vi "main-inspection-project1.vi"() -> ()   [LabVIEW 2025]
uses:
  StateVariable.ctl
panel:
  in  "stop":bool
  out "Eff (%)":dbl
  out "Part No.":i32
  out "Pass (OK)":i32
  out "MSG State":string
  out "Part result":bool
  out "Bottom Hole Pass":bool
  out "Top Hole Pass":bool
  out "Main Hole Pass":bool
  out "Distance Pass":bool
  out "Bottom Radius (Pixels)":dbl
  out "Top Radius (Pixels)":dbl
  out "Main Radius (Pixels)":dbl
  out "Distance (Clamp1)":sgl format="%.2f"
  out "appended path":path
  out "Image":T1(plugin-control)
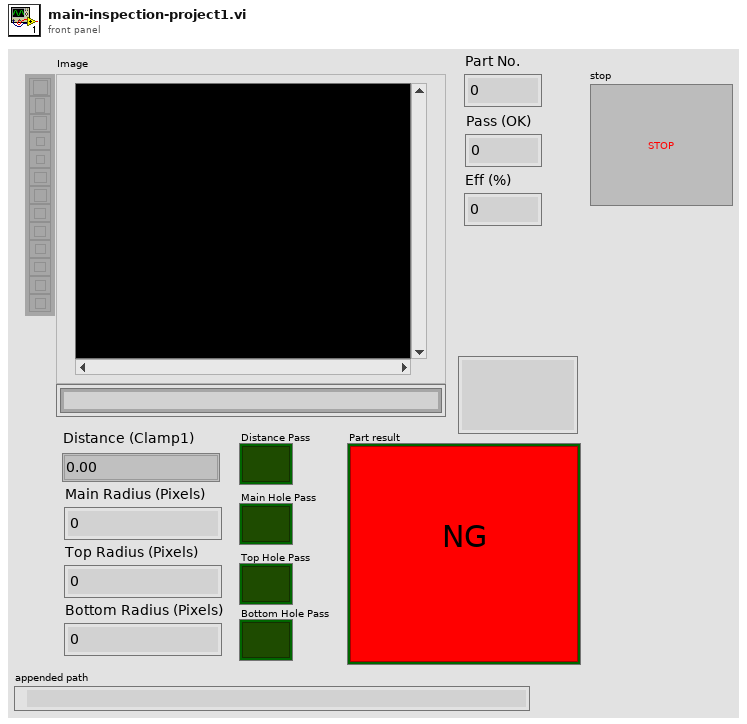
[diagram p1: front panel]
types:
  T1 = typedef "IMAQ Image.ctl" = refnum<image>
  T2 = cluster{"Distance (Clamp1)":sgl, "Main Radius (Pixels)":dbl, "Top Radius (Pixels)":dbl, "Bottom Radius (Pixels)":dbl, "Part result":bool, "Pass (OK)":i32, "PartNo.":i32, "Eff (%)":dbl, "refnum out":refnum<file>}
  T3 = typedef "StateVariable.ctl" = enum16{"Initialization", "Processing", "Checker", "Eff/Calc", "Logger", "Closed"}
  T4 = enum16{"open", "replace", "create", "open or create", "replace or create", "replace or create with confirmation"}
  T5 = cluster{"Center (Pixels)":cluster{"X":sgl, "Y":sgl}, "Radius (Pixels)":dbl, "Center (Real-World)":cluster{"X":sgl, "Y":sgl}, "Radius (Real-World)":dbl, "Roundness (Real-World)":dbl, "Average Strength":dbl, "Average SNR (dB)":dbl}
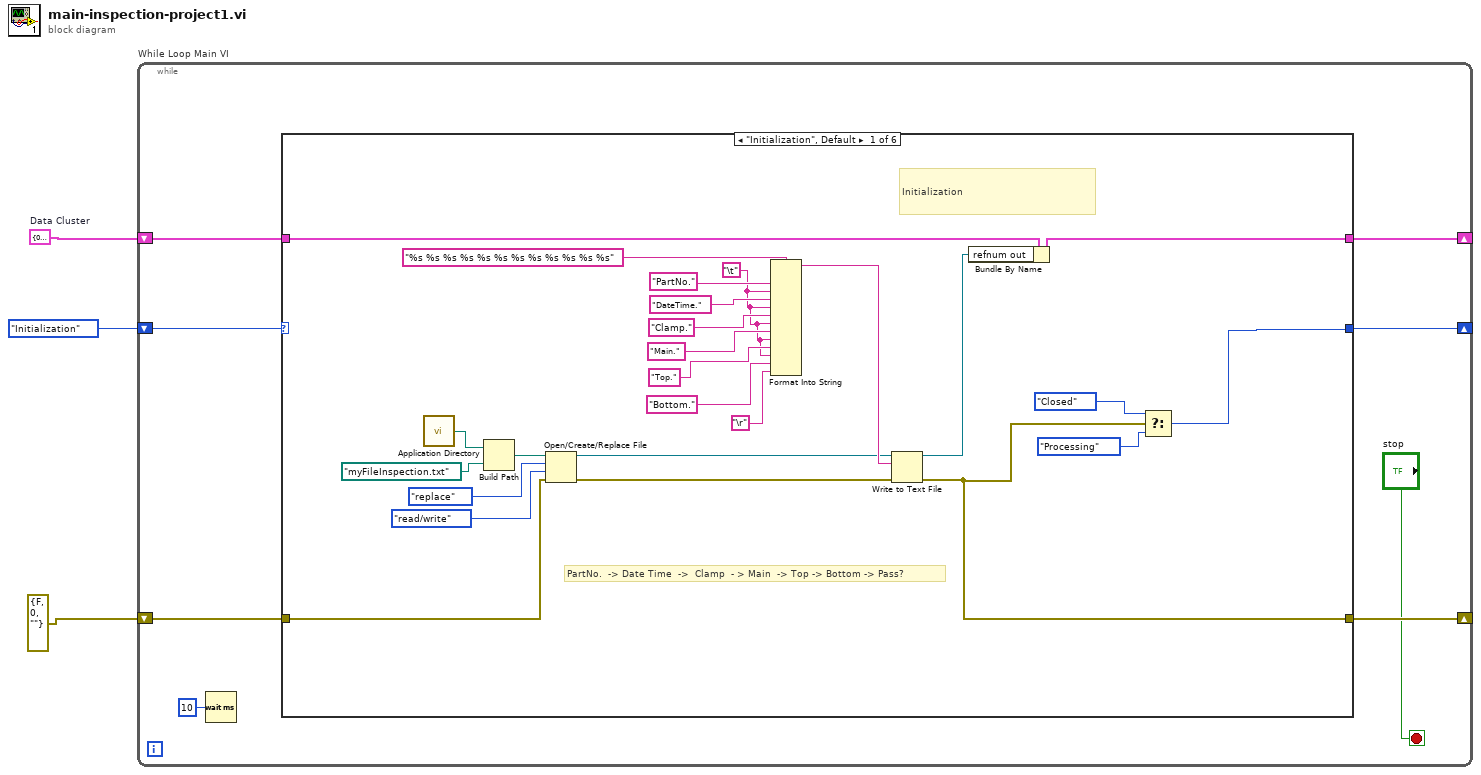
[diagram p0: block diagram]
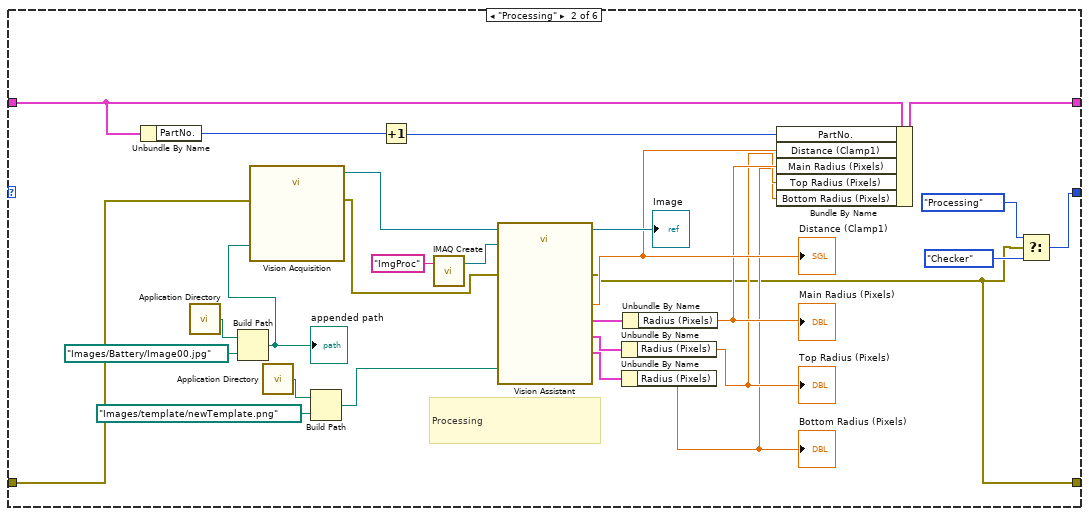
[diagram p2: hidden frame]
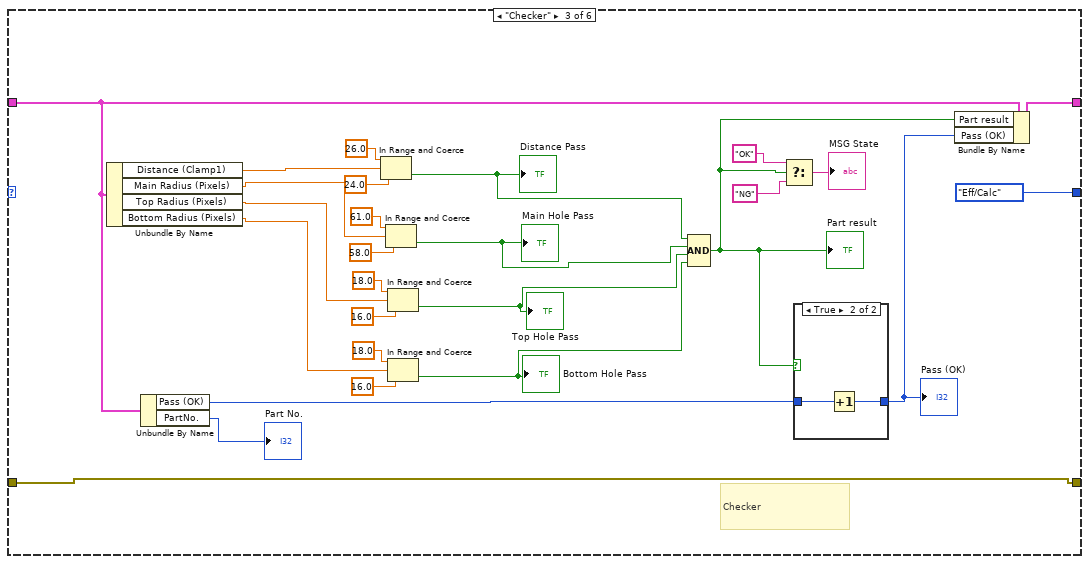
[diagram p3: hidden frame]
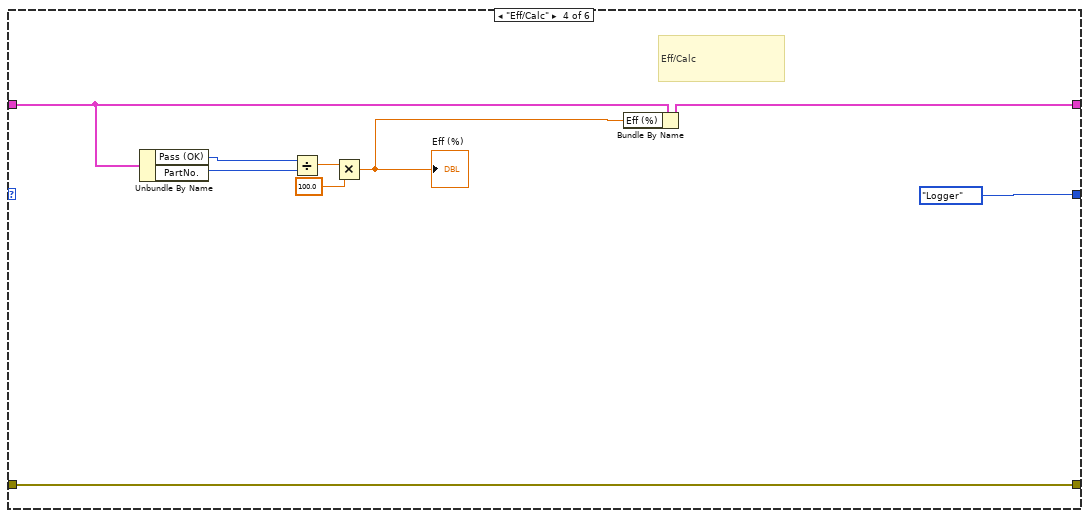
[diagram p5: hidden frame]
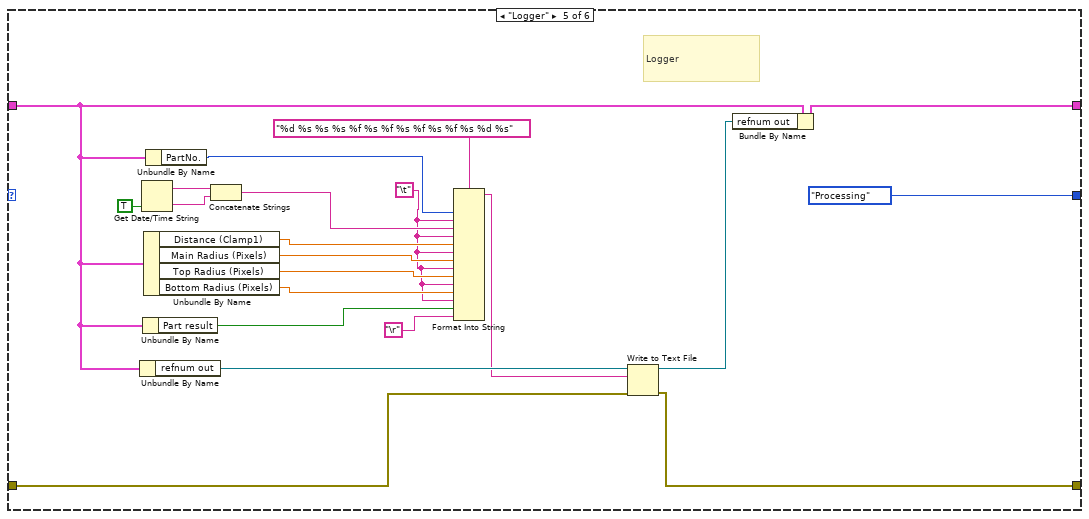
[diagram p6: hidden frame]
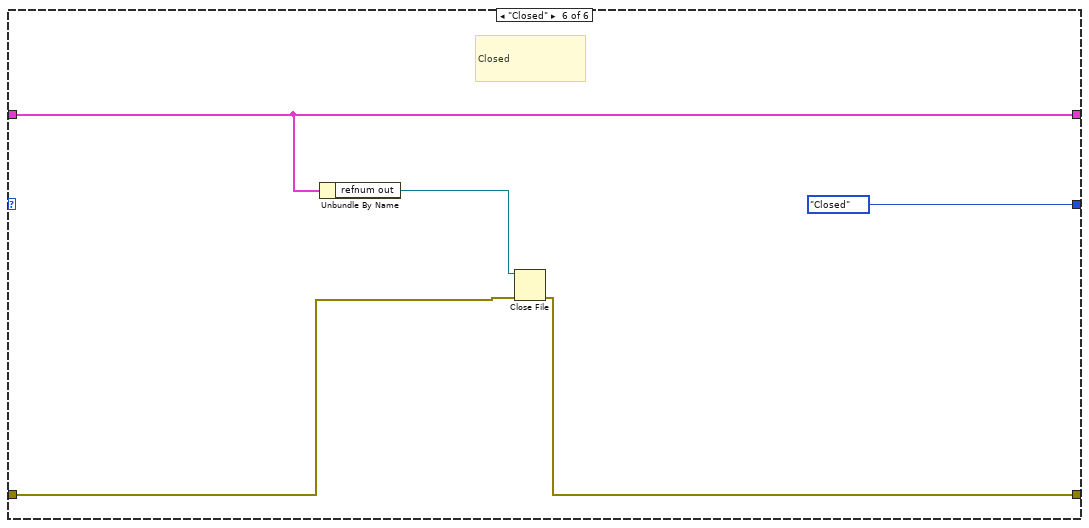
[diagram p7: hidden frame]
diagram:
  w2 = T2 {"Distance (Clamp1)"=0.0, "Main Radius (Pixels)"=0.0, "Top Radius (Pixels)"=0.0, "Bottom Radius (Pixels)"=0.0, "Part result"=FALSE, "Pass (OK)"=0, "PartNo."=0, "Eff (%)"=0.0, "refnum out"=refnum}  # Data Cluster
  n1 = while "While Loop Main VI" {
    shift-right: [w10] -> _
    shift-left: StateVariable."Initialization" ("Enum of State") -> [w11]
    shift-right: [w8] -> _
    shift-left: w2 -> [w9]
    shift-right: [w6] -> _
    shift-left: errorcluster {"status"=FALSE, "code"=0, "source"=""} ("error constant") -> [w7]
    stop <- "stop" stop-if-true
    n2 = Wait (ms)(milliseconds to wait=u32 10) -> ()  [unwired: 1 out]
    n3 = case shown="\"Initialization\", Default" w11 {
      tunnel: [w13 w40 StateVariable."Eff/Calc" ("Enum of State") StateVariable."Logger" ("Enum of State") StateVariable."Processing" ("Enum of State") StateVariable."Closed" ("Enum of State")] -> w10
      tunnel: w9 -> [w36 w39 w67 w100 w109 w127]
      tunnel: [w17 w50 w69 w95 w104 w127] -> w8
      tunnel: w7 -> [w30 w45 w89 w101 w107 w125]
      tunnel: [w14 w41 w89 w101 w106 w124] -> w6
      frame "Initialization", Default {
        w24 = "\t"
        # "PartNo.  -> Date Time  ->  Clamp  - > Main  -> Top -> Bottom -> Pass?"
        # "Initialization"
        n4 = call <vilib>:"Application Directory.vi"() -> ("Application Directory"=w35:path)
        n5 = Build Path(base path=w35, name or relative path=path "myFileInspection.txt" ("file path (use dialog)")) -> (appended path=w33:path)
        n6 = Open/Create/Replace File(file path (use dialog)=w33, error in=w30, operation (0:open)=T4."replace", access (0:read/write)=enum16{"read/write", "read-only", "write-only"}."read/write") -> (refnum out=w19:refnum<file>, error out=w18:errorcluster)  [unwired: 2 in, 1 out]
        n7 = Format Into String(format string="%s %s %s %s %s %s %s %s %s %s %s %s", "PartNo.", w24, "DateTime.", w24, "Clamp.", w24, "Main.", w24, "Top.", w24, "Bottom.", "\r") -> (resulting string=w20:string)  [unwired: 2 in, 1 out]
        n8 = Write to Text File(file (use dialog)=w19, text=w20, error in=w18) -> (refnum out=w16:refnum<file>, error out=w14:errorcluster)  [unwired: 1 in, 1 out]
        n9 = Bundle By Name(cluster=w36, "refnum out"=w16) -> (w17:T2)
        n10 = Select(t=StateVariable."Closed" ("Enum of State"), s=w14, f=StateVariable."Processing" ("Enum of State")) -> (s? t:f=w13:T3)
      }
      frame "Processing" {
        # "Processing"
        n11 = Unbundle By Name(w39) -> ("PartNo."=w38:i32)
        n12 = call <vilib>:"Application Directory.vi"() -> ("Application Directory"=w63:path)
        n13 = Build Path(base path=w63, name or relative path=path "Images/Battery/Image00.jpg") -> (appended path=w61:path)
        "appended path" <- w61
        n14 = call "Vision Acquisition"("Image Path"=w61, "error in"=w45) -> ("Image Out"=w60:T1, "error out"=w44:errorcluster)  [unwired: 22 in, 2 out]
        n15 = call <vilib>:"Application Directory.vi"() -> ("Application Directory"=w56:path)
        n16 = Build Path(base path=w56, name or relative path=path "Images/template/newTemplate.png") -> (appended path=w55:path)
        n17 = Increment(x=w38) -> (x+1=w37:i32)
        n18 = call "IMAQ Create"("Image Name"="ImgProc") -> ("New Image"=w58:T1)  [unwired: 4 in, 1 out]
        n19 = call "Vision Assistant"("Image In"=w60, "Image Dst"=w58, "Template File Path (Pattern Matching 1)"=w55, "error in"=w44) -> ("Image Out"=→"Image":T1, "Distance (Clamp1)"=w49:sgl, "Fitted Circle (Main (Hole))"=w53:T5, "Fitted Circle (Top)"=w52:T5, "Fitted Circle (Bottom)"=w51:T5, "error out"=w41:errorcluster)  [unwired: 18 in]
        "Distance (Clamp1)" <- w49
        n20 = Unbundle By Name(w52) -> ("Radius (Pixels)"=w47:dbl)
        "Top Radius (Pixels)" <- w47
        n21 = Unbundle By Name(w51) -> ("Radius (Pixels)"=w46:dbl)
        "Bottom Radius (Pixels)" <- w46
        n22 = Unbundle By Name(w53) -> ("Radius (Pixels)"=w48:dbl)
        "Main Radius (Pixels)" <- w48
        n23 = Bundle By Name(cluster=w39, "PartNo."=w37, "Distance (Clamp1)"=w49, "Main Radius (Pixels)"=w48, "Top Radius (Pixels)"=w47, "Bottom Radius (Pixels)"=w46) -> (w50:T2)
        n24 = Select(t=StateVariable."Processing" ("Enum of State"), s=w41, f=StateVariable."Checker" ("Enum of State")) -> (s? t:f=w40:T3)
      }
      frame "Checker" {
        # "Checker"
        n25 = Unbundle By Name(w67) -> ("Distance (Clamp1)"=w88:sgl, "Main Radius (Pixels)"=w83:dbl, "Top Radius (Pixels)"=w80:dbl, "Bottom Radius (Pixels)"=w78:dbl)
        n26 = Unbundle By Name(w67) -> ("Pass (OK)"=w66:i32, "PartNo."=→"Part No.":i32)
        n27 = In Range and Coerce(upper limit=sgl 26.0, x=w88, lower limit=sgl 24.0) -> (In Range?=w76:bool)  [unwired: 1 out]
        "Distance Pass" <- w76
        n28 = In Range and Coerce(upper limit=sgl 61.0, x=w83, lower limit=sgl 58.0) -> (In Range?=w75:bool)  [unwired: 1 out]
        "Main Hole Pass" <- w75
        n29 = In Range and Coerce(upper limit=sgl 18.0, x=w80, lower limit=sgl 16.0) -> (In Range?=w74:bool)  [unwired: 1 out]
        "Top Hole Pass" <- w74
        n30 = In Range and Coerce(upper limit=sgl 18.0, x=w78, lower limit=sgl 16.0) -> (In Range?=w73:bool)  [unwired: 1 out]
        "Bottom Hole Pass" <- w73
        n31 = Compound Arithmetic op=AND(w76, w75, w74, w73) -> (w68:bool)
        "Part result" <- w68
        n32 = Select(t="OK", s=w68, f="NG") -> (s? t:f=→"MSG State":string)
        n33 = case shown="True" w68 {
          tunnel: w66 -> [w91 w93]
          tunnel: [w91 w92] -> w65
          frame False {
          }
          frame True {
            n34 = Increment(x=w93) -> (x+1=w92:i32)
          }
        }
        "Pass (OK)" <- w65
        n35 = Bundle By Name(cluster=w67, "Part result"=w68, "Pass (OK)"=w65) -> (w69:T2)
      }
      frame "Eff/Calc" {
        # "Eff/Calc"
        n36 = Unbundle By Name(w100) -> ("Pass (OK)"=w99:i32, "PartNo."=w98:i32)
        n37 = Divide(x=w99, y=w98) -> (x/y=w97:dbl)
        n38 = Multiply(x=w97, y=100.0) -> (x*y=w94:dbl)
        "Eff (%)" <- w94
        n39 = Bundle By Name(cluster=w100, "Eff (%)"=w94) -> (w95:T2)
      }
      frame "Logger" {
        w113 = "\t"
        # "Logger"
        n40 = Unbundle By Name(w109) -> ("refnum out"=w108:refnum<file>)
        n41 = Get Date/Time String(want seconds? (F)=TRUE) -> (date string=w121:string, time string=w120:string)  [unwired: 2 in]
        n42 = Unbundle By Name(w109) -> ("Part result"=w112:bool)
        n43 = Unbundle By Name(w109) -> ("Distance (Clamp1)"=w117:sgl, "Main Radius (Pixels)"=w116:dbl, "Top Radius (Pixels)"=w115:dbl, "Bottom Radius (Pixels)"=w114:dbl)
        n44 = Unbundle By Name(w109) -> ("PartNo."=w119:i32)
        n45 = Concatenate Strings "Concatenate Strings"(w121, w120) -> (w118:string)
        n46 = Format Into String(format string="%d %s %s %s %f %s %f %s %f %s %f %s %d %s", w119, w113, w118, w113, w117, w113, w116, w113, w115, w113, w114, w113, w112, "\r") -> (resulting string=w105:string)  [unwired: 2 in, 1 out]
        n47 = Write to Text File(file (use dialog)=w108, text=w105, error in=w107) -> (refnum out=w103:refnum<file>, error out=w106:errorcluster)  [unwired: 1 in, 1 out]
        n48 = Bundle By Name(cluster=w109, "refnum out"=w103) -> (w104:T2)
      }
      frame "Closed" {
        # "Closed"
        n49 = Unbundle By Name(w127) -> ("refnum out"=w126:refnum<file>)
        n50 = Close File(refnum=w126, error in=w125) -> (error out=w124:errorcluster)  [unwired: 1 out]
      }
    }
  }
